vi "OpenConnection_DBL.vi"(8 "error in (no error)":errorcluster, 10 "topicName":string) -> (0 "error out":errorcluster)   [LabVIEW 2012]
uses:
  Typedefs/Control 1.ctl
panel:
  out "reference":cluster{"topicName":string, "type":refnum<vi>}
  in  "type":T1
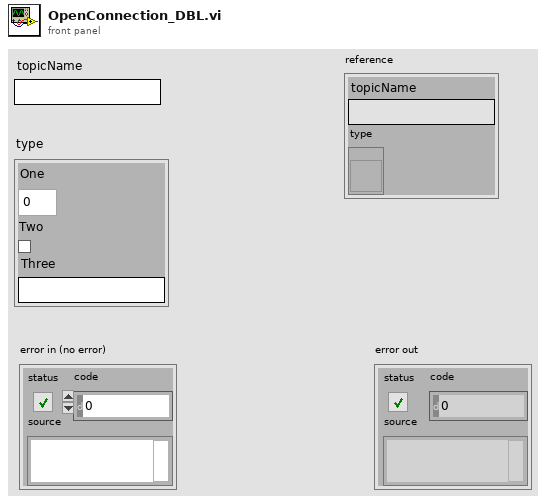
[diagram p1: front panel]
types:
  T1 = typedef "Control 1.ctl" = cluster{"One":dbl, "Two":bool, "Three":string}
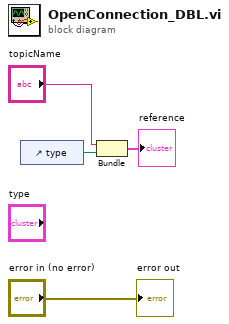
[diagram p0: block diagram]
diagram:
  n1 = control-ref of="type"() -> (w3:refnum<vi>)
  n2 = Bundle("topicName"="topicName", "type"=w3) -> (→"reference":cluster{"topicName":string, "type":refnum<vi>})  [unwired: 1 in]
  "error out" <- "error in (no error)"
